vi "CosineBasedAccelerationControl.vi"(9 "Acceleration Constant":dbl, 10 "Current Outputs":dbl[](array[numeric]), 11 "Targets":dbl[](array[numeric])) -> (3 "New Output":dbl[](array[numeric]))   [LabVIEW 2014]
panel:
  out "Loop Count":dbl[](array[numeric])
  out "Target - Current":dbl[](array[numeric])
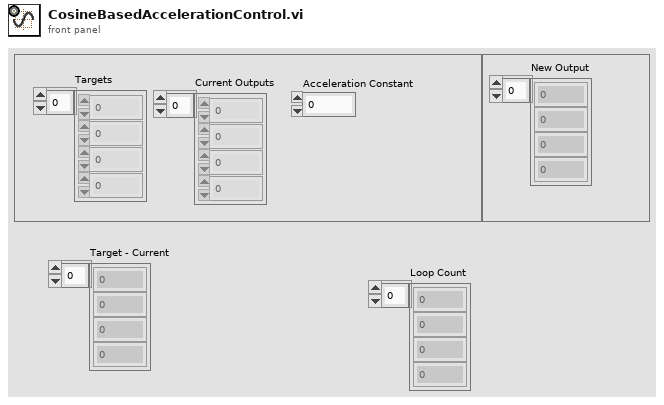
[diagram p1: front panel]
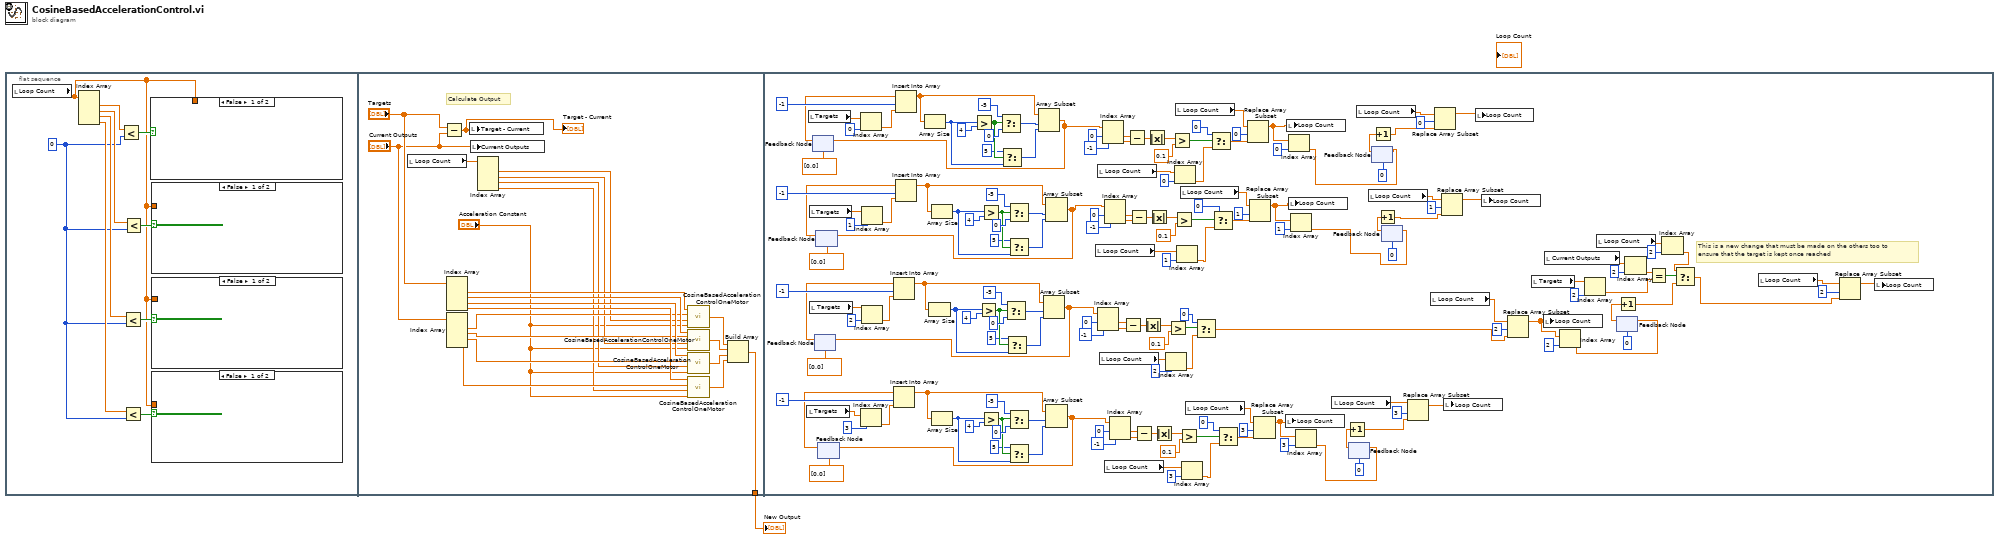
[diagram p0: block diagram]
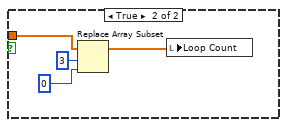
[diagram p2: hidden frame]
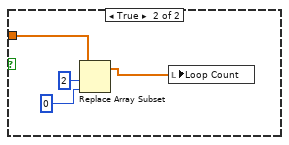
[diagram p3: hidden frame]
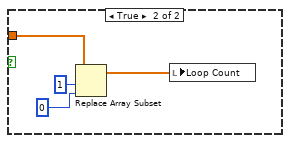
[diagram p4: hidden frame]
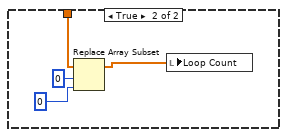
[diagram p5: hidden frame]
diagram:
  n1 = flat-sequence {
    tunnel: [w28] -> w1
    frame #0 {
      w3 = 0 ("y")
      n2 = local read "Loop Count"() -> (w2:dbl[])
      n3 = Index Array(array=w2) -> (element #1=w11:dbl, element #2=w8:dbl, element #3=w6:dbl, element #4=w4:dbl)  [unwired: 4 in]
      n4 = Less?(x=w11, y=w3) -> (x < y?=w10:bool)
      n5 = Less?(x=w6, y=w3) -> (x < y?=w7:bool)
      n6 = Less?(x=w4, y=w3) -> (x < y?=w5:bool)
      n7 = Less?(x=w8, y=w3) -> (x < y?=w9:bool)
      n8 = case shown="False" w10 {
        tunnel: w2 -> [_ w25]
        frame False {
        }
        frame True {
          n9 = Replace Array Subset(array=w25, new element=0, index=0) -> (w24:dbl[])
          n10 = local write "Loop Count"(w24) -> ()
        }
      }
      n11 = case shown="False" w9 {
        tunnel: w2 -> [_ w20]
        frame False {
        }
        frame True {
          n12 = Replace Array Subset(array=w20, new element=0, index=1) -> (w21:dbl[])
          n13 = local write "Loop Count"(w21) -> ()
        }
      }
      n14 = case shown="False" w5 {
        tunnel: w2 -> [_ w13]
        frame False {
        }
        frame True {
          n15 = Replace Array Subset(array=w13, new element=0, index=3) -> (w12:dbl[])
          n16 = local write "Loop Count"(w12) -> ()
        }
      }
      n17 = case shown="False" w7 {
        tunnel: w2 -> [_ w17]
        frame False {
        }
        frame True {
          n18 = Replace Array Subset(array=w17, new element=0, index=2) -> (w16:dbl[])
          n19 = local write "Loop Count"(w16) -> ()
        }
      }
    }
    frame #1 {
      # "Calculate Output"
      n20 = local read "Loop Count"() -> (w38:dbl[])
      n21 = Subtract(x="Targets", y="Current Outputs") -> (x-y=w49:dbl[])
      "Target - Current" <- w49
      n22 = Index Array(array="Targets") -> (element #1=w47:dbl, element #2=w46:dbl, element #3=w45:dbl, element #4=w44:dbl)  [unwired: 4 in]
      n23 = Index Array(array="Current Outputs") -> (element #1=w42:dbl, element #2=w41:dbl, element #3=w40:dbl, element #4=w39:dbl)  [unwired: 4 in]
      n24 = local write "Target - Current"(w49) -> ()
      n25 = local write "Current Outputs"("Current Outputs") -> ()
      n26 = Index Array(array=w38) -> (element #1=w37:dbl, element #2=w36:dbl, element #3=w35:dbl, element #4=w34:dbl)  [unwired: 4 in]
      n27 = call "CosineBasedAccelerationControlOneMotor.vi"("Target"=w47, "Current Output"=w42, "Loop Count"=w37, "Acceleration Scaling Constant"="Acceleration Constant") -> ("Output"=w32:dbl)  [unwired: 1 in]
      n28 = call "CosineBasedAccelerationControlOneMotor.vi"("Target"=w46, "Current Output"=w41, "Loop Count"=w36, "Acceleration Scaling Constant"="Acceleration Constant") -> ("Output"=w31:dbl)  [unwired: 1 in]
      n29 = call "CosineBasedAccelerationControlOneMotor.vi"("Target"=w45, "Current Output"=w40, "Loop Count"=w35, "Acceleration Scaling Constant"="Acceleration Constant") -> ("Output"=w30:dbl)  [unwired: 1 in]
      n30 = call "CosineBasedAccelerationControlOneMotor.vi"("Target"=w44, "Current Output"=w39, "Loop Count"=w34, "Acceleration Scaling Constant"="Acceleration Constant") -> ("Output"=w29:dbl)  [unwired: 1 in]
      n31 = Build Array(w32, w31, w30, w29) -> (w28:dbl[])
    }
    frame #2 {
      # "This is a new change that must be made on the others too to\nensure that the target is kept once reached"
      n32 = local read "Targets"() -> (w198:dbl[])
      n33 = local read "Targets"() -> (w217:dbl[])
      n34 = local read "Targets"() -> (w210:dbl[])
      n35 = local read "Targets"() -> (w204:dbl[])
      n36 = feedback #1(dbl[] [0.0]) -> (w214:dbl[])
      n37 = feedback #2(dbl[] [0.0]) -> (w203:dbl[])
      n38 = feedback #3(dbl[] [0.0]) -> (w208:dbl[])
      n39 = feedback #4(dbl[] [0.0]) -> (w196:dbl[])
      n40 = Index Array(array=w217, index=0) -> (element=w215:dbl)
      n41 = Index Array(array=w198, index=3) -> (element=w199:dbl)
      n42 = Index Array(array=w210, index=1) -> (element=w211:dbl)
      n43 = Index Array(array=w204, index=2) -> (element=w206:dbl)
      n44 = Insert Into Array(array=w203, index=-1, new element=w206) -> (w168:dbl[])
      n45 = Insert Into Array(array=w196, index=-1, new element=w199) -> (w159:dbl[])
      n46 = Insert Into Array(array=w214, index=-1, new element=w215) -> (w186:dbl[])
      n47 = Insert Into Array(array=w208, index=-1, new element=w211) -> (w177:dbl[])
      n48 = Array Size(array=w186) -> (size(s)=w187:i32)
      n49 = Array Size(array=w168) -> (size(s)=w169:i32)
      n50 = Array Size(array=w177) -> (size(s)=w178:i32)
      n51 = Array Size(array=w159) -> (size(s)=w160:i32)
      n52 = Greater?(x=w187, y=4) -> (0:w190:bool)
      n53 = Greater?(x=w169, y=4) -> (0:w172:bool)
      n54 = Greater?(x=w178, y=4) -> (0:w181:bool)
      n55 = Greater?(x=w160, y=4) -> (0:w163:bool)
      n56 = Select(t=-5, s=w190, f=0) -> (s? t:f=w194:i32)
      n57 = Select(t=5, s=w190, f=w187) -> (s? t:f=w188:i32)
      n58 = Select(t=-5, s=w172, f=0) -> (s? t:f=w176:i32)
      n59 = Select(t=5, s=w172, f=w169) -> (s? t:f=w170:i32)
      n60 = Select(t=-5, s=w181, f=0) -> (s? t:f=w185:i32)
      n61 = Select(t=-5, s=w163, f=0) -> (s? t:f=w167:i32)
      n62 = Select(t=5, s=w181, f=w178) -> (s? t:f=w179:i32)
      n63 = Select(t=5, s=w163, f=w160) -> (s? t:f=w161:i32)
      n64 = Array Subset(array=w186, index=w194, length=w188) -> (w66:dbl[])
      n65 = feedback-in #1(w66) -> ()
      n66 = Array Subset(array=w168, index=w176, length=w170) -> (w156:dbl[])
      n67 = feedback-in #2(w156) -> ()
      n68 = Array Subset(array=w177, index=w185, length=w179) -> (w112:dbl[])
      n69 = feedback-in #3(w112) -> ()
      n70 = Array Subset(array=w159, index=w167, length=w161) -> (w74:dbl[])
      n71 = feedback-in #4(w74) -> ()
      n72 = local read "Loop Count"() -> (w69:dbl[])
      n73 = Index Array(array=w156, index #1=0 ("index"), index #2=-1 ("index")) -> (element #1=w154:dbl, element #2=w155:dbl)
      n74 = local read "Loop Count"() -> (w64:dbl[])
      n75 = local read "Loop Count"() -> (w124:dbl[])
      n76 = Index Array(array=w66, index #1=0 ("index"), index #2=-1 ("index")) -> (element #1=w98:dbl, element #2=w97:dbl)
      n77 = Index Array(array=w112, index #1=0 ("index"), index #2=-1 ("index")) -> (element #1=w114:dbl, element #2=w113:dbl)
      n78 = local read "Loop Count"() -> (w72:dbl[])
      n79 = Index Array(array=w74, index #1=0 ("index"), index #2=-1 ("index")) -> (element #1=w83:dbl, element #2=w82:dbl)
      n80 = Subtract(x=w155, y=w154) -> (x-y=w153:dbl)
      n81 = Subtract(x=w98, y=w97) -> (x-y=w101:dbl)
      n82 = Subtract(x=w114, y=w113) -> (x-y=w117:dbl)
      n83 = Subtract(x=w83, y=w82) -> (x-y=w86:dbl)
      n84 = Absolute Value(x=w153) -> (abs(x)=w152:dbl)
      n85 = Absolute Value(x=w101) -> (abs(x)=w100:dbl)
      n86 = Absolute Value(x=w117) -> (abs(x)=w116:dbl)
      n87 = Absolute Value(x=w86) -> (abs(x)=w85:dbl)
      n88 = Index Array(array=w124, index=2) -> (element=w122:dbl)
      n89 = Greater?(x=w152, y=0.1) -> (0:w150:bool)
      n90 = Greater?(x=w100, y=0.1) -> (0:w95:bool)
      n91 = Greater?(x=w116, y=0.1) -> (0:w110:bool)
      n92 = Index Array(array=w64, index=0) -> (element=w94:dbl)
      n93 = local read "Loop Count"() -> (w65:dbl[])
      n94 = Index Array(array=w69, index=1) -> (element=w109:dbl)
      n95 = Greater?(x=w85, y=0.1) -> (0:w80:bool)
      n96 = local read "Loop Count"() -> (w67:dbl[])
      n97 = Index Array(array=w72, index=3) -> (element=w79:dbl)
      n98 = local read "Loop Count"() -> (w71:dbl[])
      n99 = Select(t=0, s=w150, f=w122) -> (s? t:f=w125:dbl)
      n100 = Select(t=0, s=w95, f=w94) -> (s? t:f=w92:dbl)
      n101 = Select(t=0, s=w110, f=w109) -> (s? t:f=w107:dbl)
      n102 = Select(t=0, s=w80, f=w79) -> (s? t:f=w77:dbl)
      n103 = Replace Array Subset(array=w65, new element=w92, index=0) -> (w63:dbl[])
      n104 = Replace Array Subset(array=w67, new element=w107, index=1) -> (w68:dbl[])
      n105 = Replace Array Subset(array=w71, new element=w77, index=3) -> (w70:dbl[])
      n106 = local write "Loop Count"(w70) -> ()
      n107 = local write "Loop Count"(w63) -> ()
      n108 = Index Array(array=w63, index=0) -> (element=w89:dbl)
      n109 = local write "Loop Count"(w68) -> ()
      n110 = Index Array(array=w68, index=1) -> (element=w104:dbl)
      n111 = Index Array(array=w70, index=3) -> (element=w73:dbl)
      n112 = local read "Loop Count"() -> (w133:dbl[])
      n113 = feedback-in #5(w73) -> ()
      n114 = feedback #5(0) -> (w130:dbl)
      n115 = Increment(x=w130) -> (x+1=w129:dbl)
      n116 = local read "Loop Count"() -> (w148:dbl[])
      n117 = local read "Loop Count"() -> (w144:dbl[])
      n118 = feedback #6(0) -> (w220:dbl)
      n119 = feedback-in #6(w89) -> ()
      n120 = Increment(x=w220) -> (x+1=w145:dbl)
      n121 = feedback-in #7(w104) -> ()
      n122 = feedback #7(0) -> (w141:dbl)
      n123 = Increment(x=w141) -> (x+1=w139:dbl)
      n124 = Replace Array Subset(array=w133, new element=w129, index=3) -> (w128:dbl[])
      n125 = local read "Loop Count"() -> (w127:dbl[])
      n126 = Replace Array Subset(array=w148, new element=w145, index=0) -> (w146:dbl[])
      n127 = Replace Array Subset(array=w144, new element=w139, index=1) -> (w143:dbl[])
      n128 = local write "Loop Count"(w128) -> ()
      n129 = local write "Loop Count"(w146) -> ()
      n130 = local write "Loop Count"(w143) -> ()
      n131 = Replace Array Subset(array=w127, new element=w125, index=2) -> (w62:dbl[])
      n132 = local read "Targets"() -> (w57:dbl[])
      n133 = local write "Loop Count"(w62) -> ()
      n134 = local read "Current Outputs"() -> (w61:dbl[])
      n135 = Index Array(array=w62, index=2) -> (element=w120:dbl)
      n136 = Index Array(array=w57, index=2) -> (element=w56:dbl)
      n137 = local read "Loop Count"() -> (w53:dbl[])
      n138 = feedback-in #8(w120) -> ()
      n139 = feedback #8(0) -> (w134:dbl)
      n140 = Increment(x=w134) -> (x+1=w54:dbl)
      n141 = Index Array(array=w61, index=2) -> (element=w59:dbl)
      n142 = Equal?(x=w59, y=w56) -> (x = y?=w55:bool)
      n143 = Index Array(array=w53, index=2) -> (element=w51:dbl)
      n144 = Select(t=w51, s=w55, f=w54) -> (s? t:f=w50:dbl)
      n145 = local read "Loop Count"() -> (w138:dbl[])
      n146 = Replace Array Subset(array=w138, new element=w50, index=2) -> (w137:dbl[])
      n147 = local write "Loop Count"(w137) -> ()
    }
  }
  "New Output" <- w1
